vi "USSTest.vi"() -> ()   [LabVIEW 2019]
uses:
  WSCbot_V3_Toolkit.lvlibp
panel:
  out "Waveform Chart":dbl(graph)
  in  "Stop Button":bool
  out "Distance_R(mm)":dbl
  out "Distance_L(mm)":dbl
  out "error out":errorcluster
  in  "Enable_R":bool=TRUE
  in  "Enable_L":bool=TRUE
  in  "error in":errorcluster
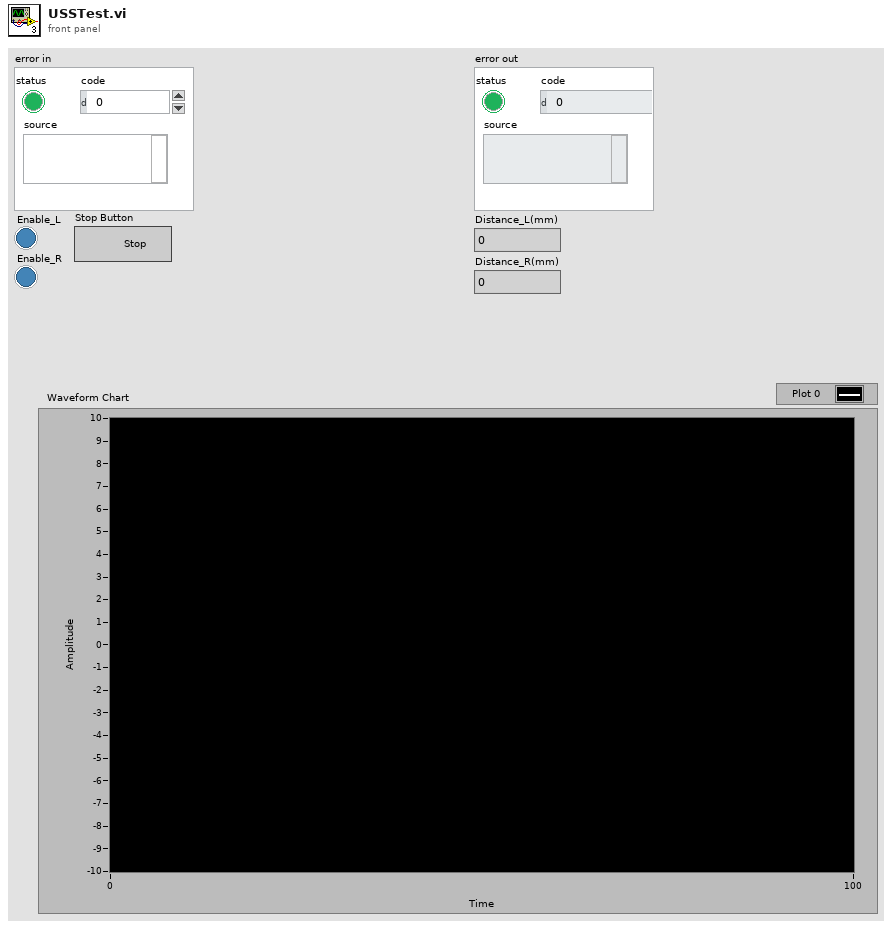
[diagram p1: front panel]
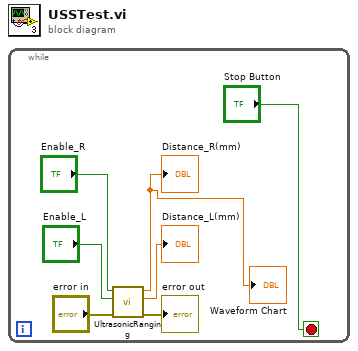
[diagram p0: block diagram]
diagram:
  n1 = while {
    stop <- "Stop Button" stop-if-true
    n2 = call "UltrasonicRanging.vi"("error in"="error in", "Enable_L"="Enable_L", "Enable_R"="Enable_R") -> ("error out"=→"error out":errorcluster, "Distance_L(mm)"=→"Distance_L(mm)":dbl, "Distance_R(mm)"=→"Distance_R(mm)" →"Waveform Chart":dbl)  [unwired: 6 in]
  }
